vi "FGV_DB.vi"(0 "HGF_FGV_Action":refnum<class "HGF_FGV_Action.lvclass">, 5 "error in (no error)":errorcluster) -> (14 "dup HGF_FGV_Action":refnum<class "HGF_FGV_Action.lvclass">, 19 "error out":errorcluster)   [LabVIEW 2012, in "HGF_FGV.lvlib"]
doc: "This VI is a Functional Global Variable that contains an array of LabVIEW objects. The object array is cleared on first call.\n\nThe objects can be accessed by appling anHGF_FGV_Action that contains the Object index it should be applied to and the concrete action.\n\n<B>Attention:</B> This FGV is reentrant! So it should not be used explicity, but it should be called from a non-reentrant VI that represents an individual FGV database instance."
uses:
  HGF_FGV.lvlib
  HGF_FGV_Action/HGF_FGV_Action.lvclass
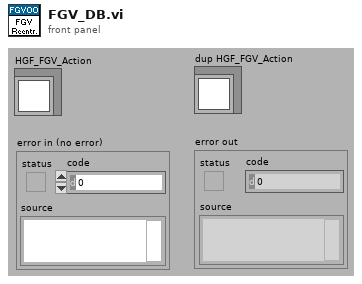
[diagram p1: front panel]
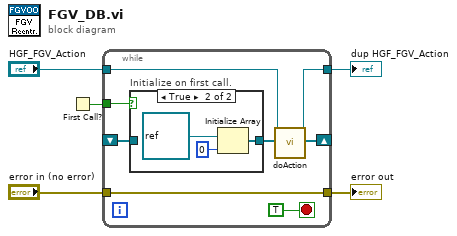
[diagram p0: block diagram]
diagram:
  n1 = First Call?() -> (First Call?: T/F=w1:bool)
  n2 = while {
    tunnel: "HGF_FGV_Action" -> [w11]
    tunnel: [w10] -> w4
    tunnel: "error in (no error)" -> [w13]
    tunnel: [w13] -> w2
    tunnel: w1 -> [w9]
    shift-right: [w7] -> _
    shift-left: _ -> [w6]
    stop <- TRUE stop-if-true
    n3 = case "Initialize on first call." shown="True" w9 {
      tunnel: w6 -> [w14 _]
      tunnel: [w14 w16] -> w8
      frame False {
      }
      frame True {
        n4 = Initialize Array(refnum<class> refnum ("LabVIEW Object"), 0 ("dimension size")) -> (w16:refnum<class>[])
      }
    }
    n5 = call "doAction.vi"("HGF_FGV_Action"=w11, "Objects"=w8) -> ("dup HGF_FGV_Action"=w10:refnum<class "HGF_FGV_Action.lvclass">, "dup Objects"=w7:refnum<class>[])  [unwired: 1 in, 15 out]
  }
  "dup HGF_FGV_Action" <- w4
  "error out" <- w2
